vi "Append (double array).vi"(6 "Reset":bool, 8 "error in (no error)":errorcluster, 9 "Y-array":dbl[](array[numeric]), 10 "X-array":dbl[](array[numeric]), 11 "XY-data (A)":cluster{"X-array":dbl[], "Y-array":dbl[]}) -> (0 "error out":errorcluster, 3 "XY-data out":cluster{"X-array":dbl[], "Y-array":dbl[]} {"Y-array" format="%.2p"; "X-array" format="%.2p"})   [LabVIEW 2019, in "xy_utilities.lvlib"]
doc: "Append <B>XY-Data B</B> to the end of <B>XY-Data A</B> (similar to Append Waveforms.vi).\n\nWire data to the data input to determine the polymorphic instance to use or manually select the instance."
uses:
  xy_utilities.lvlib
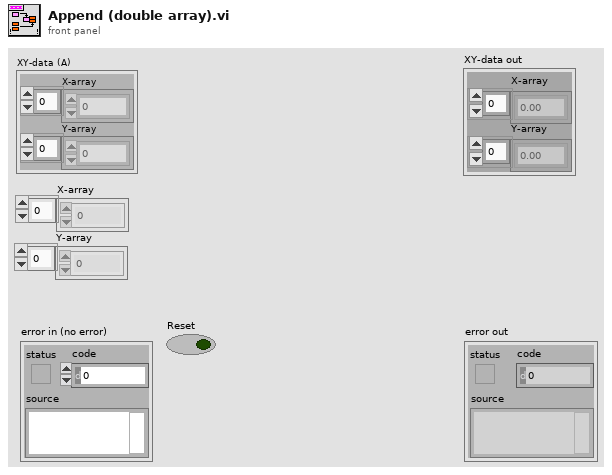
[diagram p1: front panel]
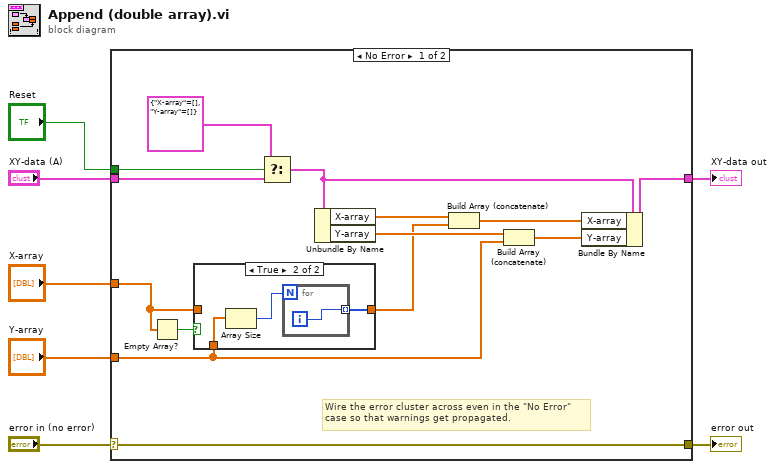
[diagram p0: block diagram]
diagram:
  n1 = case shown="No Error" "error in (no error)" {
    selector: "error in (no error)" -> [w21 w28]
    tunnel: [w21 w28] -> w6
    tunnel: "XY-data (A)" -> [w14 w27]
    tunnel: [w20 w27] -> w4
    tunnel: "X-array" -> [w9 _]
    tunnel: "Y-array" -> [w8 _]
    tunnel: "Reset" -> [w15 _]
    frame No Error {
      # "Wire the error cluster across even in the \"No Error\"\ncase so that warnings get propagated."
      n2 = Empty Array?(array=w9) -> (empty?=w11:bool)
      n3 = case shown="True" w11 {
        tunnel: [w22 w25] -> w10
        tunnel: w9 -> [w22 _]
        tunnel: w8 -> [_ w24]
        frame False {
        }
        frame True {
          n4 = Array Size(array=w24) -> (size(s)=w23:i32)
          n5 = for {
            N: w23 -> [_]
            tunnel: [w26] -> w25 mode=indexing
            i -> [w26]
          }
        }
      }
      n6 = Select(t=cluster{"X-array":dbl[], "Y-array":dbl[]} {"X-array"=[], "Y-array"=[]} ("XY-data (A)"), s=w15, f=w14) -> (s? t:f=w13:cluster{"X-array":dbl[], "Y-array":dbl[]})
      n7 = Unbundle By Name(w13) -> ("X-array"=w19:dbl[], "Y-array"=w17:dbl[])
      n8 = Build Array (concatenate)(w19, w10) -> (w18:dbl[])
      n9 = Build Array (concatenate)(w17, w8) -> (w16:dbl[])
      n10 = Bundle By Name(cluster=w13, "X-array"=w18, "Y-array"=w16) -> (w20:cluster{"X-array":dbl[], "Y-array":dbl[]})
    }
    frame Error {
    }
  }
  "error out" <- w6
  "XY-data out" <- w4
